vi "AssetInterface_Initalize Assets.vi"(8 "error in (no error)":errorcluster, 11 "EnergyStorage in":refnum<class "EnergyStorage.lvclass">) -> (0 "error out":errorcluster, 2 "TagDescriptions":refnum<class "tag descriptor.lvclass">[](array[class]), 3 "EnergyStorage out":refnum<class "EnergyStorage.lvclass">)   [LabVIEW 2015, in "EnergyStorage.lvclass"]
uses:
  EnergyStorage.lvclass
  <vilib>/NI/Tag Bus/tag/tag descriptor.lvclass
  TagBus/TagBus.lvclass
panel:
  out "EnergyStorage_Control":cluster{"kW setpoint":dbl}
  out "EnergyStorage_Status":cluster{"kW":dbl}
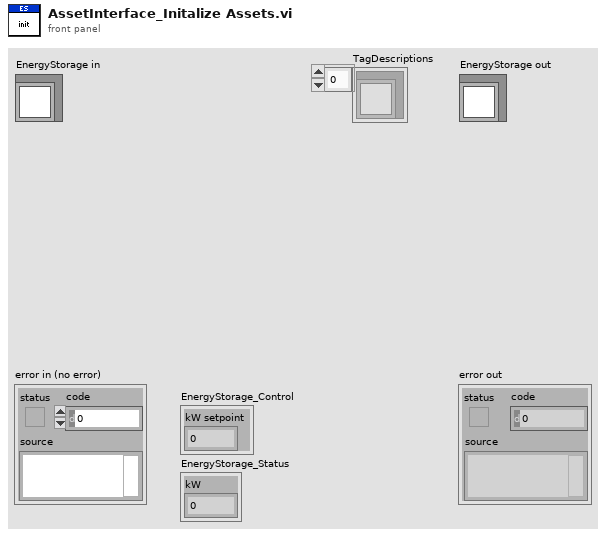
[diagram p1: front panel]
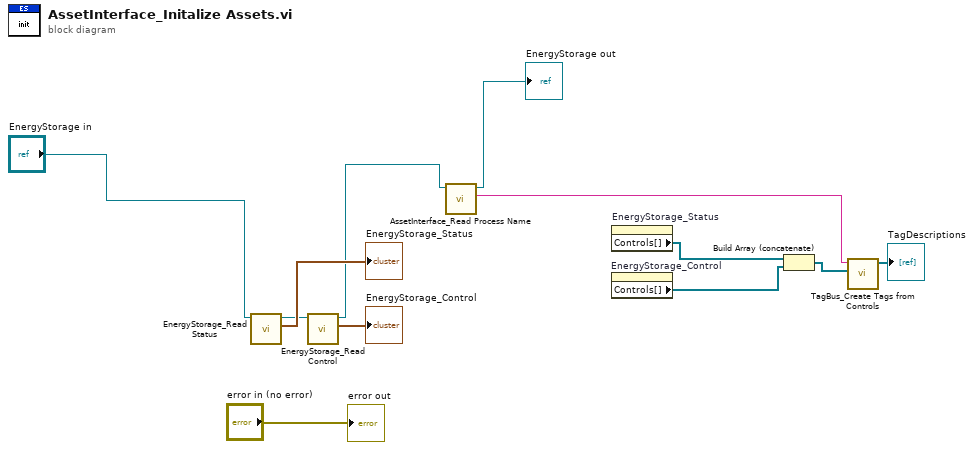
[diagram p0: block diagram]
diagram:
  n1 = call-dynamic "EnergyStorage_Read Status.vi"("EnergyStorage in"="EnergyStorage in") -> ("EnergyStorage_Status"=→"EnergyStorage_Status":cluster{"kW":dbl}, "EnergyStorage out"=w11:refnum<class "EnergyStorage.lvclass">)  [unwired: 9 in]
  n2 = call-dynamic "EnergyStorage_Read Control.vi"("EnergyStorage in"=w11) -> ("EnergyStorage_Control"=→"EnergyStorage_Control":cluster{"kW setpoint":dbl}, "EnergyStorage out"=w5:refnum<class "EnergyStorage.lvclass">)  [unwired: 9 in]
  n3 = call-dynamic "AssetInterface_Read Process Name.vi"("EnergyStorage in"=w5) -> ("Process Name"=w3:string, "EnergyStorage out"=→"EnergyStorage out":refnum<class "EnergyStorage.lvclass">)  [unwired: 9 in]
  n4 = property on="EnergyStorage_Status" class="Clust (strict)"() -> ("Controls[]"=w7:refnum<vi>[])  [unwired: 2 in, 2 out]
  n5 = property on="EnergyStorage_Control" class="Clust (strict)"() -> ("Controls[]"=w6:refnum<vi>[])  [unwired: 2 in, 2 out]
  n6 = Build Array (concatenate)(w7, w6) -> (w2:refnum<vi>[])
  n7 = call "TagBus_Create Tags from Controls.vi"("Array"=w2, "Process Name"=w3) -> ("TagDescriptions"=→"TagDescriptions":refnum<class "tag descriptor.lvclass">[])  [unwired: 9 in]
  "error out" <- "error in (no error)"
